vi "Behaviour on Error on Input.vi"() -> ()   [LabVIEW 2017]
uses:
  HSE-Logger/Handler/LokiHandler/LokiHandler.lvclass
  C:/Projects/HSE Logger/Source/HSE-Logger/Handler/Handler.lvclass
  HSE-Logger/hse-logger.lvlib
panel:
  out "ijk":errorcluster
  out "ghi":errorcluster
  out "efg":errorcluster
  out "cde":errorcluster
  out "abc":errorcluster
  in  "error in":errorcluster
  # "See block diagram\nfor explanation..."
  # "Locals"
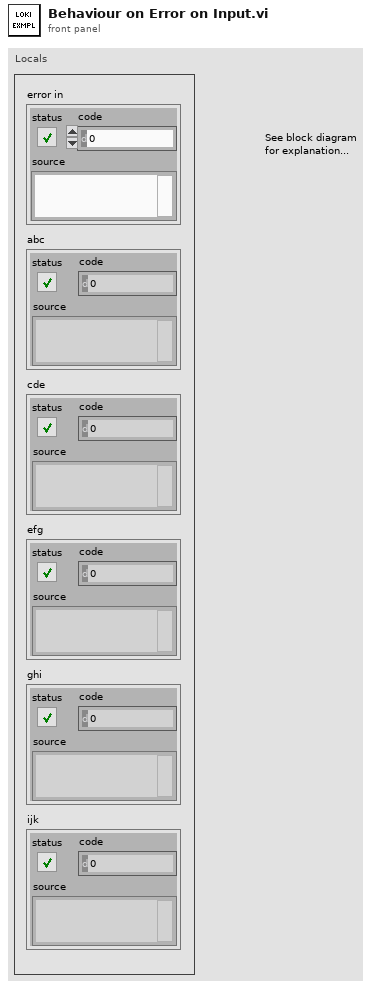
[diagram p1: front panel]
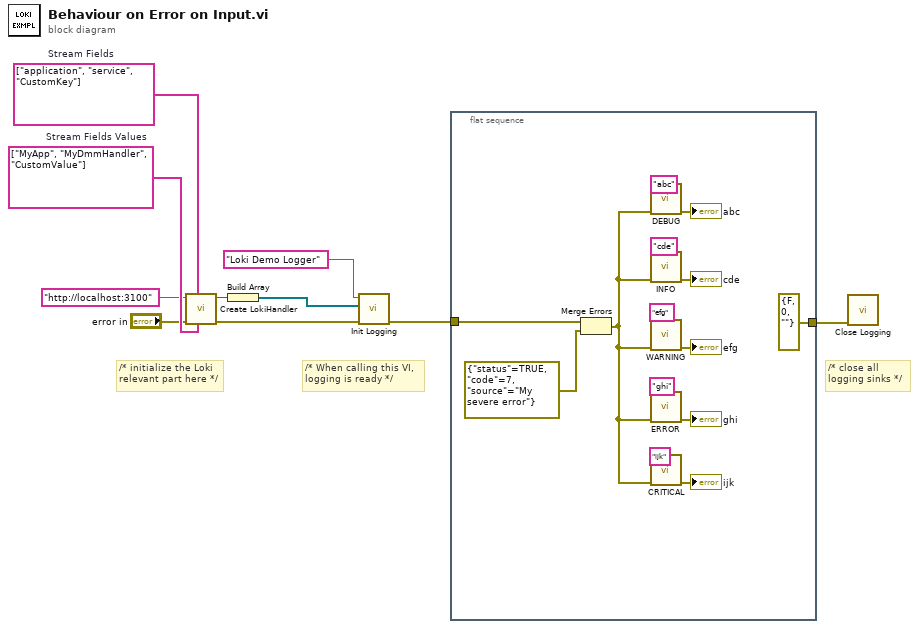
[diagram p0: block diagram]
diagram:
  w7 = string[] ["MyApp", "MyDmmHandler", "CustomValue"]  # Stream Fields Values
  w6 = string[] ["application", "service", "CustomKey"]  # Stream Fields
  # "/* close all \nlogging sinks */"
  # "/* When calling this VI,\nlogging is ready */"
  # "/* initialize the Loki\nrelevant part here */"
  n1 = call "Create LokiHandler.vi"("Stream Fields Values"=w7, "Stream Fields"=w6, "error in"="error in", "Loki URL and Port"="http://localhost:3100") -> ("error out"=w3:errorcluster, "LokiHandler out"=w10:refnum<class "LokiHandler.lvclass">)  [unwired: 6 in]
  n2 = Build Array(w10) -> (w9:refnum<class "LokiHandler.lvclass">[])
  n3 = call "Init Logging.vi"("error in"=w3, "Handlers"=w9, "Name"="Loki Demo Logger") -> ("error out"=w2:errorcluster)  [unwired: 8 in]
  n4 = flat-sequence {
    tunnel: w2 -> [w18]
    tunnel: [errorcluster {"status"=FALSE, "code"=0, "source"=""} ("error out")] -> w1
    frame #0 {
      n5 = Merge Errors(w18, errorcluster {"status"=TRUE, "code"=7, "source"="My severe error"} ("error in")) -> (w17:errorcluster)
      n6 = call "DEBUG.vi"("Message"="abc", "error in"=w17) -> ("error out"=→"abc":errorcluster)  [unwired: 9 in]
      n7 = call "INFO.vi"("Message"="cde", "error in"=w17) -> ("error out"=→"cde":errorcluster)  [unwired: 9 in]
      n8 = call "WARNING.vi"("Message"="efg", "error in"=w17) -> ("error out"=→"efg":errorcluster)  [unwired: 9 in]
      n9 = call "ERROR.vi"("Message"="ghi", "error in"=w17) -> ("error out"=→"ghi":errorcluster)  [unwired: 9 in]
      n10 = call "CRITICAL.vi"("Message"="ijk", "error in"=w17) -> ("error out"=→"ijk":errorcluster)  [unwired: 9 in]
    }
  }
  n11 = call "Close Logging.vi"("error in"=w1) -> ()  [unwired: 10 in, 1 out]
